vi "ShiftRegister.vi"() -> ()   [LabVIEW 2022 SP3]
panel:
  out "Numeric 7":dbl
  out "Numeric 6":dbl
  out "Numeric 5":dbl
  out "Numeric 4":dbl
  out "Numeric 3":i32
  out "Numeric 2":dbl
  out "Numeric":i32
  out "x+y":i32
  out "Array 2":dbl[](array[numeric])
  out "number: 0 to 2":dbl
  out "number: 0 to 1":dbl
  out "Array":dbl[](array[numeric])
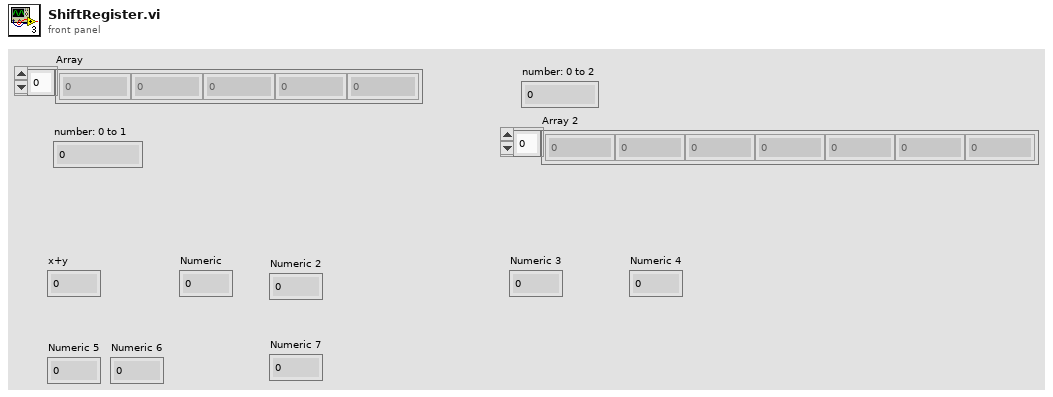
[diagram p1: front panel]
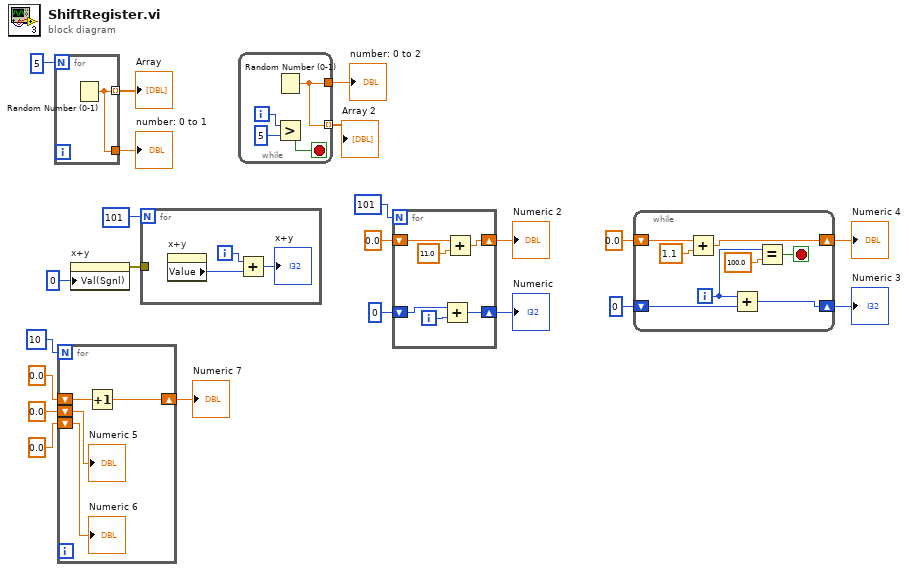
[diagram p0: block diagram]
diagram:
  n1 = for {
    N: 5 -> [_]
    tunnel: [w23] -> w21 mode=indexing
    tunnel: [w23] -> w20
    n2 = Random Number (0-1)() -> (number: 0 to 1=w23:dbl)
  }
  "Array" <- w21
  "number: 0 to 1" <- w20
  n3 = for {
    N: 10 -> [_]
    shift-right: [w27] -> w1
    shift-left: 0.0 -> [w26]
    shift-left: 0.0 -> [w25]
    shift-left: 0.0 -> [w24]
    n4 = Increment(x=w26) -> (x+1=w27:dbl)
    "Numeric 5" <- w25
    "Numeric 6" <- w24
  }
  "Numeric 7" <- w1
  n5 = property on="x+y" class="DigNum (strict)"("Val(Sgnl)"=0 ("Value (Signaling)")) -> (error out=w15:errorcluster)  [unwired: 2 in, 1 out]
  n6 = for {
    N: 101 -> [_]
    tunnel: w15 -> [_]
    i -> [w30]
    n7 = property on="x+y" class="DigNum (strict)"() -> ("Value"=w28:i32)  [unwired: 2 in, 2 out]
    n8 = Add(x=w30, y=w28) -> (x+y=→"x+y":i32)
  }
  n9 = while {
    tunnel: [w31] -> w19
    tunnel: [w31] -> w18 mode=indexing
    i -> [w34]
    stop <- w32 stop-if-true
    n10 = Random Number (0-1)() -> (number: 0 to 1=w31:dbl)
    n11 = Greater?(x=w34, y=5) -> (0:w32:bool)
  }
  "number: 0 to 2" <- w19
  "Array 2" <- w18
  n12 = for {
    N: 101 -> [_]
    shift-right: [w39] -> w14
    shift-left: 0 -> [w38]
    shift-right: [w36] -> w10
    shift-left: 0.0 -> [w35]
    i -> [w40]
    n13 = Add(x=w38, y=w40) -> (x+y=w39:i32)
    n14 = Add(x=w35, y=11.0) -> (x+y=w36:dbl)
  }
  "Numeric" <- w14
  "Numeric 2" <- w10
  n15 = while {
    shift-right: [w48] -> w8
    shift-left: 0 -> [w44]
    shift-right: [w42] -> w6
    shift-left: 0.0 -> [w43]
    i -> [w45]
    stop <- w46 stop-if-true
    n16 = Add(x=w43, y=1.1) -> (x+y=w42:dbl)
    n17 = Add(x=w45, y=w44) -> (x+y=w48:i32)
    n18 = Equal?(x=w45, y=100.0) -> (x = y?=w46:bool)
  }
  "Numeric 3" <- w8
  "Numeric 4" <- w6
